vi "Generate Random Numbers.vi"(8 "random numbers per second":dbl, 9 "stop length":i32, 10 "elapsed time":dbl, 11 "current array size":i32) -> (2 "done?":bool, 3 "random numbers out":dbl[](array[numeric]))   [LabVIEW 2020, in "Service.lvlib"]
uses:
  Service.lvlib
  <vilib>/numeric/Random Number (Range) DBL.vi
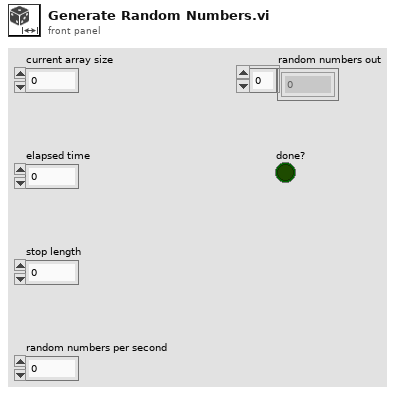
[diagram p1: front panel]
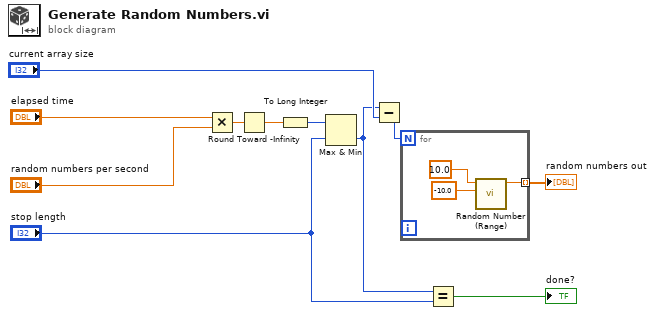
[diagram p0: block diagram]
diagram:
  n1 = Multiply(x="elapsed time", y="random numbers per second") -> (x*y=w10:dbl)
  n2 = Round Toward -Infinity(1:w10) -> (0:w9:dbl)
  n3 = To Long Integer(number=w9) -> (32bit integer=w6:i32)
  n4 = Max & Min(x=w6, y="stop length") -> (min(x,y)=w3:i32)  [unwired: 1 out]
  n5 = Subtract(x=w3, y="current array size") -> (x-y=w4:i32)
  n6 = for {
    N: w4 -> [_]
    tunnel: [w12] -> w11 mode=indexing
    n7 = call-poly <vilib>:"Random Number (Range).vi"("lower bound (0)"=-10.0, "upper bound (100)"=10.0) -> ("number"=w12:dbl)  [unwired: 9 in]
  }
  "random numbers out" <- w11
  n8 = Equal?(x=w3, y="stop length") -> (x = y?=→"done?":bool)
